vi "Read Lossy.vi"(0 "Wait for Next? (F)":bool, 2 "FlexChannel":T2, 3 "Wait Timeout mS (-1)":i32=-1) -> (5 "Updated":timestamp, 6 "Timed Out?":bool, 7 "Value":T1, 8 "New Value?":bool, 9 "Closed?":bool)   [LabVIEW 2022 SP3, in "Flex.lvlib"]
doc: "Allows reading tag-like data from the channel. This reader endpoint will behave closer to a notifier if the <b>Wait for Next</b> input is set to true otherwise it will return the latest value that has been set. The Timeout will only apply when Wait for Next is set. The <b>Closed</b> output will return true when the writer has been closed and can be used to close down the reader's loop."
uses:
  Flex.lvlib
  ))Channel.ctl
  Element.ctl
  ChannelOp.ctl
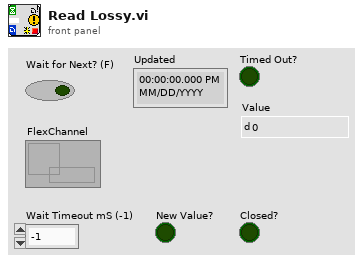
[diagram p1: front panel]
types:
  T1 = typedef "Flex.lvlib/Element.ctl" = dbl
  T2 = typedef "Flex.lvlib/))Channel.ctl" = refnum<queue>
  T3 = typedef "Flex.lvlib/ChannelOp.ctl" = enum16{"Get Refs", "Init", "Close", "Probe", "New Queue", "Remove Queue", "New Event"}
  T4 = typedef "Flex.lvlib/Channel Data.ctl" = cluster{"Event":refnum<user-event>, "Writer Ref":refnum<data-value>, "Lossy Queue":refnum<queue>, "Update":refnum<k4>}
  T5 = typedef "Flex.lvlib/Element Info.ctl" = cluster{"Value":T1, "Updated":timestamp, "Sequence":u32, "Paused":bool}
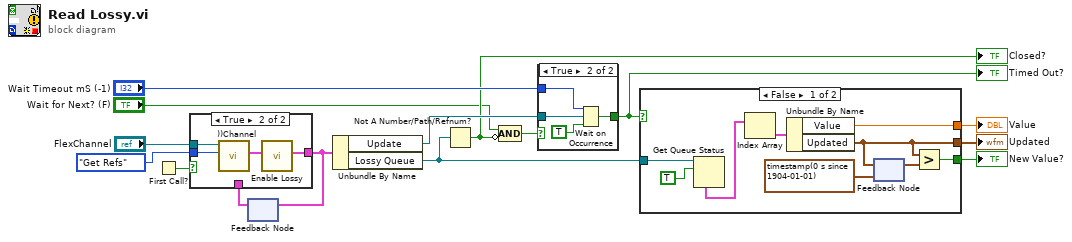
[diagram p0: block diagram]
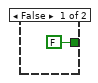
[diagram p3: hidden frame]
diagram:
  n1 = First Call?() -> (First Call?: T/F=w13:bool)
  n2 = feedback #1() -> (w12:T4)  [unwired: 1 in]
  n3 = case shown="True" w13 {
    tunnel: "FlexChannel" -> [_ w20]
    tunnel: ChannelOp."Get Refs" ("channelOp") -> [_ w19]
    tunnel: [w16 w17] -> w10
    tunnel: w12 -> [w16 _]
    frame False {
    }
    frame True {
      n4 = call "))Channel.vi"("channelOp"=w19, "channel in"=w20) -> ("Channel Data"=w18:T4)  [unwired: 5 in, 4 out]
      n5 = call "Enable Lossy.vi"("Channel Data In"=w18) -> ("Channel Data"=w17:T4)  [unwired: 10 in]
    }
  }
  n6 = feedback-in #1(w10) -> ()
  n7 = Unbundle By Name(w10) -> ("Update"=w7:refnum<k4>, "Lossy Queue"=w4:refnum<queue>)
  n8 = Not A Number/Path/Refnum?(number/path/refnum=w4) -> (NaN/Path/Refnum?=w3:bool)
  "Closed?" <- w3
  n9 = Compound Arithmetic op=AND("Wait for Next? (F)", invert w3) -> (w1:bool)
  n10 = case shown="True" w1 {
    tunnel: w7 -> [_ w24]
    tunnel: "Wait Timeout mS (-1)" -> [_ w23]
    tunnel: [FALSE ("timed out") w22] -> w5
    frame False {
    }
    frame True {
      n11 = Wait on Occurrence(1:TRUE ("ignore previous (T)"), 2:w24, 3:w23) -> (0:w22:bool)
    }
  }
  "Timed Out?" <- w5
  n12 = case shown="False" w5 {
    tunnel: [w34 _] -> w11
    tunnel: w4 -> [w33 _]
    tunnel: [w32 _] -> w9
    tunnel: [w31 _] -> w8
    frame False {
      n13 = Get Queue Status(queue=w33, return elements? (F)=TRUE) -> (elements=w29:T5[])  [unwired: 1 in, 7 out]
      n14 = Index Array(array=w29) -> (element=w28:T5)  [unwired: 1 in]
      n15 = Unbundle By Name(w28) -> ("Value"=w34:T1, "Updated"=w32:timestamp)
      n16 = feedback #2(timestamp(0 s since 1904-01-01) ("Updated")) -> (w26:timestamp)
      n17 = feedback-in #2(w32) -> ()
      n18 = Greater?(x=w32, y=w26) -> (0:w31:bool)
    }
    frame True {
    }
  }
  "Value" <- w11
  "Updated" <- w9
  "New Value?" <- w8
